vi "CM-Read Display Settings.vi"(0 "configuration file path":path=path "C:/PXI Connections.txt", 11 "error in (no error)":errorcluster) -> (4 "file path":path, 15 "error out":errorcluster)   [LabVIEW 2015]
uses:
  <vilib>/Utility/config.llb/NI_LVConfig.lvlib
  <vilib>/Utility/config.llb/Read Key (Boolean).vi
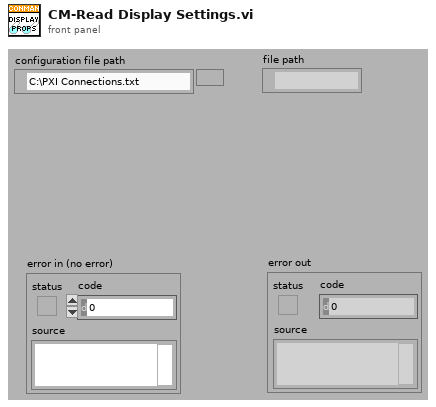
[diagram p1: front panel]
types:
  T1 = typedef "NI_LVConfig.lvlib/Config Data RefNum.ctl" = refnum<k1>
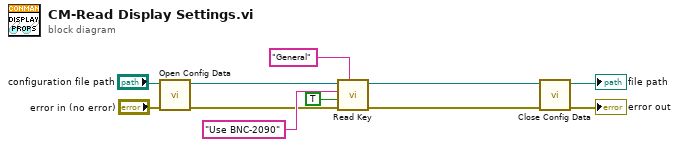
[diagram p0: block diagram]
diagram:
  n1 = call <vilib>:"Open Config Data.vi"("error in (no error)"="error in (no error)", "configuration file path"="configuration file path") -> ("error out"=w3:errorcluster, "refnum"=w4:T1)  [unwired: 7 in, 1 out]
  n2 = call-poly <vilib>:"Read Key.vi"("section"="General", "error in (no error)"=w3, "default value"=TRUE, "key"="Use BNC-2090", "refnum"=w4) -> ("error out"=w7:errorcluster, "refnum out"=w6:T1)  [unwired: 3 in, 2 out]
  n3 = call <vilib>:"Close Config Data.vi"("error in (no error)"=w7, "refnum"=w6) -> ("error out"=→"error out":errorcluster, "file path"=→"file path":path)  [unwired: 8 in]
